vi "Write Message (UDP).vi"(4 "address":cluster{"address":u32, "port":u16}, 6 "options":T1={"ignore timeout error"=TRUE, "timeout ms (1000)"=1000}, 8 "error in":errorcluster, 9 "data":string, 10 "name":string, 11 "connection info in":T2) -> (0 "error out":errorcluster, 3 "connection info out":T2)   [LabVIEW 2013, in "NI STM.lvlib"]
doc: "This VI writes a package of data to a remote computer. It prepends a meta data ID number to each packet. \n\nThe data must be passed in as a String. The calling VI is responsible for flattening the desired data to a string before passing it to this VI."
uses:
  NI STM.lvlib
  UDP Connection Info.ctl
  SubVIs/MetaDataElement.ctl
  UDP Write Options.ctl
  SubVIs/GetIDfromName.vi
  SubVIs/Generate Error.vi
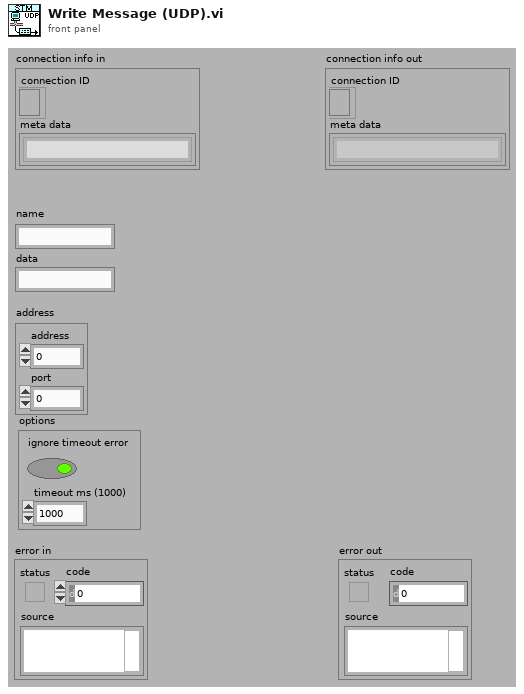
[diagram p1: front panel]
types:
  T1 = typedef "NI STM.lvlib/UDP Write Options.ctl" = cluster{"ignore timeout error":bool, "timeout ms (1000)":i32}
  T2 = typedef "NI STM.lvlib/UDP Connection Info.ctl" = cluster{"connection ID":refnum<k16>, "meta data":T3[]}
  T3 = typedef "NI STM.lvlib/MetaDataElement.ctl" = string
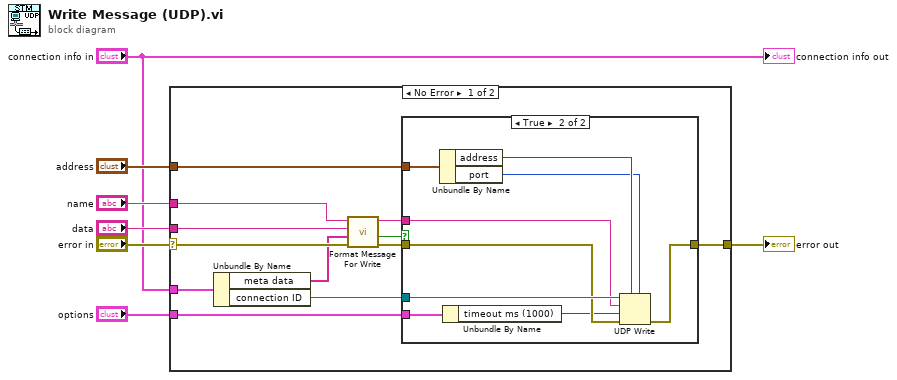
[diagram p0: block diagram]
diagram:
  n1 = case shown="No Error" "error in" {
    selector: "error in" -> [w16 w30]
    tunnel: "connection info in" -> [w17 _]
    tunnel: [w19 w30] -> w7
    tunnel: "name" -> [w14 _]
    tunnel: "data" -> [w13 _]
    tunnel: "address" -> [w8 _]
    tunnel: "options" -> [w9 _]
    frame No Error {
      n2 = Unbundle By Name(w17) -> ("meta data"=w12:T3[], "connection ID"=w18:refnum<k16>)
      n3 = call "Format Message For Write.vi"("error in"=w16, "meta data"=w12, "data"=w13, "message name"=w14) -> ("error out"=w15:errorcluster, "valid?"=w11:bool, "message"=w10:string)  [unwired: 5 in]
      n4 = case shown="True" w11 {
        tunnel: w18 -> [_ w28]
        tunnel: w15 -> [w20 w26]
        tunnel: [w20 w29] -> w19
        tunnel: w10 -> [_ w27]
        tunnel: w9 -> [_ w24]
        tunnel: w8 -> [_ w21]
        frame False {
        }
        frame True {
          n5 = Unbundle By Name(w21) -> ("address"=w23:u32, "port"=w22:u16)
          n6 = Unbundle By Name(w24) -> ("timeout ms (1000)"=w25:i32)
          n7 = UDP Write(address=w23, port or service name=w22, connection ID=w28, data in=w27, 8:w26, 9:w25) -> (error out=w29:errorcluster)  [unwired: 1 out]
        }
      }
    }
    frame Error {
    }
  }
  "error out" <- w7
  "connection info out" <- "connection info in"
